vi "Model Status To OPCUA.vi"(8 "error in (no error)":errorcluster, 11 "Model_AMC in":refnum<class "Model_AMC.lvclass">) -> (0 "error out":errorcluster, 3 "Model_AMC out":refnum<class "Model_AMC.lvclass">)   [LabVIEW 2021, in "Model_AMC.lvclass"]
uses:
  Model_AMC.lvclass
  Model_AMC.lvclass/Model_AMC.ctl
  <userlib>/John_Lib/OPCUA/OPCUA.lvclass
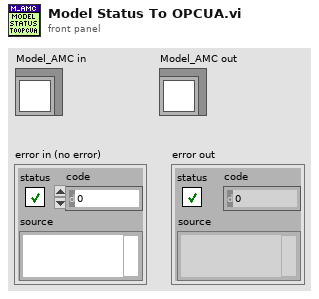
[diagram p1: front panel]
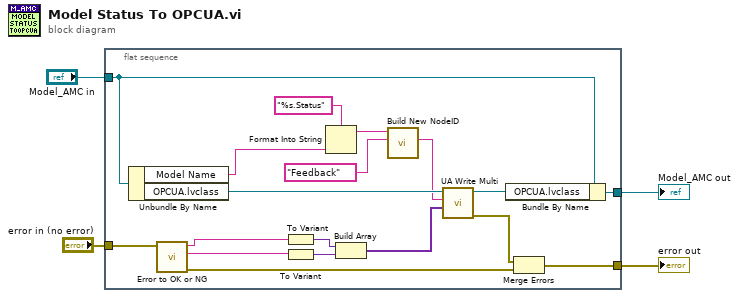
[diagram p0: block diagram]
diagram:
  n1 = flat-sequence {
    tunnel: "Model_AMC in" -> [w21]
    tunnel: [w20] -> w3
    tunnel: [w19] -> w2
    tunnel: "error in (no error)" -> [w6]
    frame #0 {
      n2 = Unbundle By Name(w21) -> ("Model Name"=w7:string, "OPCUA.lvclass"=w18:refnum<class "OPCUA.lvclass">)
      n3 = call <userlib>:"Error to OK or NG.vi"("error in (no error)"=w6) -> ("error out"=w5:errorcluster, "Error source"=w13:string, "OK/NG"=w14:string)  [unwired: 7 in, 1 out]
      n4 = To Variant(anything=w14) -> (Variant=w12:variant)
      n5 = To Variant(anything=w13) -> (Variant=w11:variant)
      n6 = Format Into String(format string="%s.Status" ("node ID"), w7) -> (resulting string=w17:string)  [unwired: 2 in, 1 out]
      n7 = Build Array(w12, w11) -> (w10:variant[])
      n8 = call <userlib>:"Build New NodeID.vi"("SubName"="Feedback", "node ID"=w17) -> ("NodeIDs Old and New"=w15:string)  [unwired: 6 in, 3 out]
      n9 = call <userlib>:"UA Write Multi.vi"("ValueArray"=w10, "node IDs"=w15, "OPCUA in"=w18) -> ("error out"=w8:errorcluster, "OPCUA out"=w9:refnum<class "OPCUA.lvclass">)  [unwired: 6 in, 1 out]
      n10 = Bundle By Name(cluster=w21, "OPCUA.lvclass"=w9) -> (w20:refnum<class "Model_AMC.lvclass">)
      n11 = Merge Errors(w8, w5) -> (w19:errorcluster)
    }
  }
  "error out" <- w2
  "Model_AMC out" <- w3
